vi "After Write.vi"(8 "error in":errorcluster, 9 "State In":variant, 10 "Compiled Settings":variant, 11 "Custom Device API in":refnum<class "Custom Device API.lvclass">) -> (0 "error out":errorcluster, 1 "State Out":variant, 3 "Custom Device API out":refnum<class "Custom Device API.lvclass">)   [LabVIEW 2026, in "Template Test Hooks.lvlib"]
uses:
  Template Test Hooks.lvlib
  <userlib>/Custom Device Interfaces_v1.lvlibp/CustomDeviceAPI/Custom Device API.lvclass
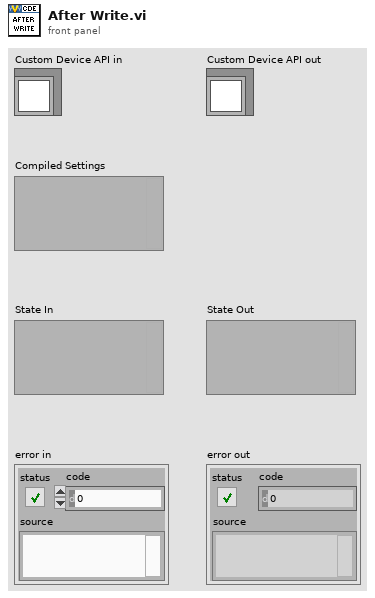
[diagram p1: front panel]
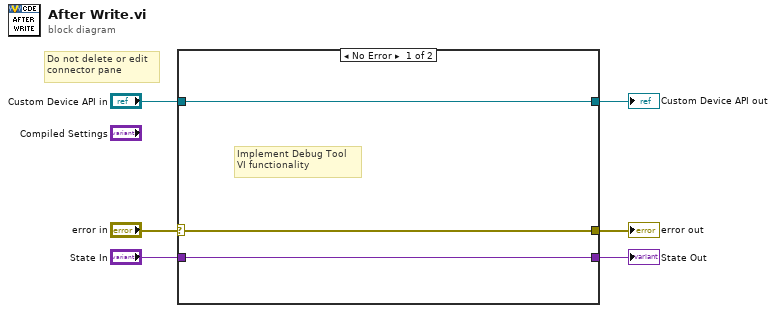
[diagram p0: block diagram]
diagram:
  # "Do not delete or edit \nconnector pane"
  n1 = case shown="No Error" "error in" {
    selector: "error in" -> [w9 w11]
    tunnel: [w9 w11] -> w5
    tunnel: "Custom Device API in" -> [w8 w12]
    tunnel: [w8 w12] -> w3
    tunnel: "State In" -> [w7 w10]
    tunnel: [w7 w10] -> w1
    frame No Error {
      # "Implement Debug Tool\nVI functionality"
    }
    frame Error {
    }
  }
  "Custom Device API out" <- w3
  "error out" <- w5
  "State Out" <- w1
